vi "Read Item Symbols.vi"(8 "error in (no error)":errorcluster, 11 "Tree in":refnum<class "Tree.lvclass">) -> (0 "error out":errorcluster, 2 "Item Symbols":dbl[](array[numeric]) format="%#_f", 3 "Tree out":refnum<class "Tree.lvclass">)   [LabVIEW 2019, in "Tree.lvclass"]
uses:
  Tree.lvclass
  Tree.lvclass/Tree.ctl
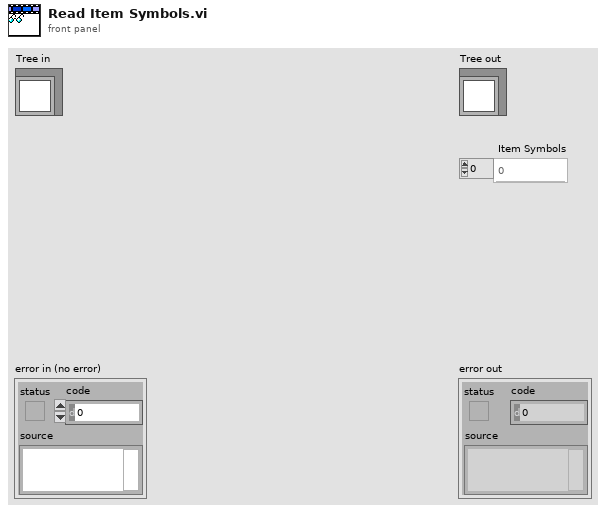
[diagram p1: front panel]
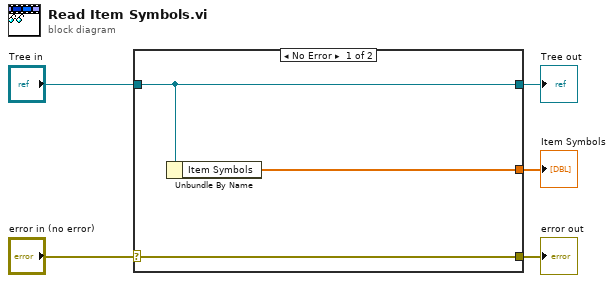
[diagram p0: block diagram]
diagram:
  n1 = case shown="No Error" "error in (no error)" {
    selector: "error in (no error)" -> [w8 w9]
    tunnel: [w8 w9] -> w4
    tunnel: [w7 w10] -> w2
    tunnel: "Tree in" -> [w7 w10]
    tunnel: [w6 _] -> w1
    frame No Error {
      n2 = Unbundle By Name(w7) -> ("Item Symbols"=w6:dbl[])
    }
    frame Error {
    }
  }
  "error out" <- w4
  "Tree out" <- w2
  "Item Symbols" <- w1
